vi "Create TCP Slave.vi"(8 "error in":errorcluster, 9 "device data model":refnum<class "Device Data Model.lvclass">, 10 "port (502)":u16=502) -> (0 "error out":errorcluster, 3 "TCP slave instance":refnum<class "Modbus Slave.lvclass">)   [LabVIEW 2015, in "Modbus Library.lvlib" / "API Main.lvlib"]
doc: "Creates a standard TCP slave with an IP ADU. If the data model input is unwired, a standard data model will be initialized and used. If the input is wired, the code will check to make sure that it is not the default value for the class (it should be initialized). If the default value of the class is wired, the standard model will be initialized and used."
uses:
  API Main.lvlib
  Slave/Modbus Slave.lvclass
  Data Model/Device Data Model.lvclass
  Transmission Data Unit/IP/IP Data Unit.lvclass
  Network Protocol/Network Slave/TCP/TCP Slave.lvclass
  Transmission Data Unit/Transmission Data Unit.lvclass/Transmission Data Unit.ctl
  Network Protocol/Network Slave/TCP/TCP Slave.lvclass/TCP Slave.ctl
  Standard Data Model/Standard Data Model.lvclass
  Data Model/Device Data Model.lvclass/Device Data Model.ctl
  Slave/Modbus Slave.lvclass/Modbus Slave.ctl
  Modbus API.lvclass/Modbus API.ctl
  Network Protocol/Network Slave/TCP/Write Port.vi
  Data Model/Read Initialized.vi
  <vilib>/Utility/error.llb/Clear Errors.vi
  Modbus API.lvclass
  Transmission Data Unit/Transmission Data Unit.lvclass
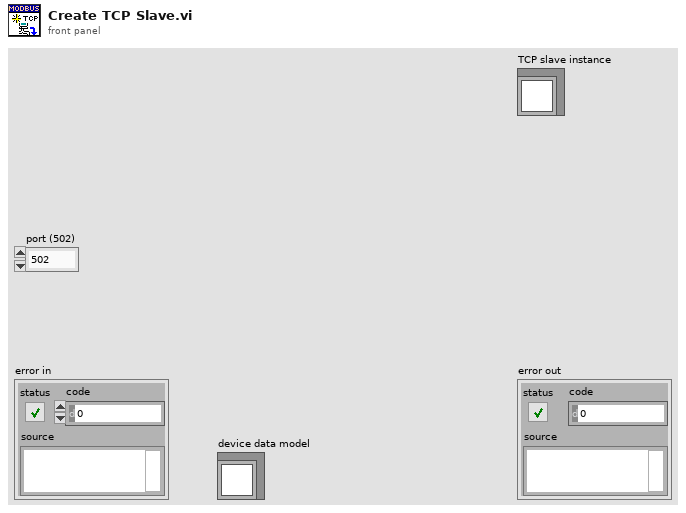
[diagram p1: front panel]
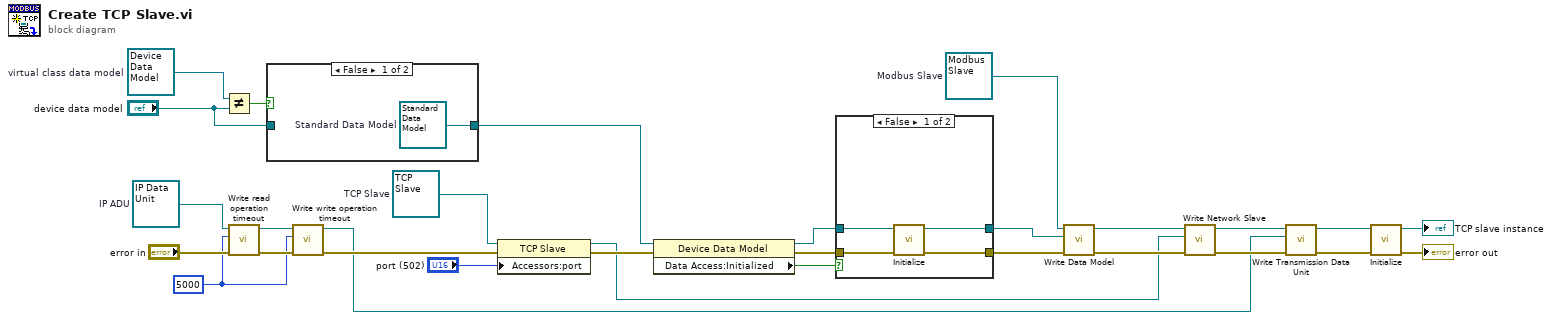
[diagram p0: block diagram]
diagram:
  w21 = refnum<class "Device Data Model.lvclass"> refnum  # virtual class data model
  w2 = 5000 ("read operation timeout")
  w29 = refnum<class "TCP Slave.lvclass"> refnum  # TCP Slave
  w4 = refnum<class "IP Data Unit.lvclass"> refnum  # IP ADU
  w15 = refnum<class "Modbus Slave.lvclass"> refnum  # Modbus Slave
  n1 = Not Equal?(x=w21, y="device data model") -> (x != y?=w20:bool)
  n2 = call "Write read operation timeout.vi"("error in (no error)"="error in", "read operation timeout"=w2, "transmission data unit in"=w4) -> ("error out"=w6:errorcluster, "transmission data unit out"=w3:refnum<class "IP Data Unit.lvclass">)  [unwired: 7 in]
  n3 = case shown="False" w20 {
    tunnel: "device data model" -> [_ w31]
    tunnel: [w30 w31] -> w18
    frame False {
      w30 = refnum<class "Standard Data Model.lvclass"> refnum  # Standard Data Model
    }
    frame True {
    }
  }
  n4 = call "Write write operation timeout.vi"("error in (no error)"=w6, "write operation timeout"=w2, "transmission data unit in"=w3) -> ("error out"=w7:errorcluster, "transmission data unit out"=w1:refnum<class "IP Data Unit.lvclass">)  [unwired: 7 in]
  n5 = property class="TCP Slave"(reference=w29, error in=w7, "Accessors:port"="port (502)") -> (reference out=w8:refnum<class "TCP Slave.lvclass">, error out=w25:errorcluster)
  n6 = property class="Device Data Model"(reference=w18, error in=w25) -> (reference out=w23:refnum<class "Device Data Model.lvclass">, error out=w24:errorcluster, "Data Access:Initialized"=w22:bool)
  n7 = case shown="False" w22 {
    tunnel: w24 -> [w35 w37]
    tunnel: [w34 w37] -> w16
    tunnel: [w33 w36] -> w17
    tunnel: w23 -> [w32 w36]
    frame False {
      n8 = call-dynamic "Initialize.vi"("error in"=w35, "device data model in"=w32) -> ("error out"=w34:errorcluster, "device data model out"=w33:refnum<class "Device Data Model.lvclass">)  [unwired: 8 in]
    }
    frame True {
    }
  }
  n9 = call "Write Data Model.vi"("error in"=w16, "Device Data Model"=w17, "Modbus slave in"=w15) -> ("error out"=w9:errorcluster, "Modbus slave out"=w11:refnum<class "Modbus Slave.lvclass">)  [unwired: 7 in]
  n10 = call "Write Network Slave.vi"("error in"=w9, "network slave"=w8, "Modbus slave in"=w11) -> ("error out"=w10:errorcluster, "Modbus slave out"=w12:refnum<class "Modbus Slave.lvclass">)  [unwired: 7 in]
  n11 = call "Write Transmission Data Unit.vi"("error in"=w10, "transmission data unit"=w1, "Modbus instance in"=w12) -> ("error out"=w13:errorcluster, "Modbus instance out"=w14:refnum<class "Modbus Slave.lvclass">)  [unwired: 7 in]
  n12 = call-dynamic "Initialize.vi"("error in"=w13, "Modbus slave in"=w14) -> ("error out"=→"error out":errorcluster, "Modbus slave out"=→"TCP slave instance":refnum<class "Modbus Slave.lvclass">)  [unwired: 8 in]
